vi "Init Message Transport Data Binding.vi"(8 "error in (no error)":errorcluster, 9 "Control Indexes":i32[](array[numeric]), 10 "VI Refnum":refnum<vi>) -> (0 "error out":errorcluster, 3 "Message Transport Binding out":refnum<class "Message Transport Binding.lvclass">)   [LabVIEW 2016, in "Stream Mediator.lvlib" / "Message Transport Binding.lvclass"]
doc: "--\nCopyright © 2017 Composed SystemsI All rights reserved.\n\nAuthor: Jon McBee <jon.mcbee@composed.io>\n\nThis library is provided \"AS IS\" ,WITHOUT WARRANTIES OR\nCONDITIONS OF ANY KIND, either express or implied.\n\nComposed Systems -- composed.io\n\nStream 0.0.1.1\nJon McBee - Composed Systems\nCopyright (c) 2017, Composed Systems"
uses:
  <userlib>/Composed Systems/Stream/Mediator/Classes/Message Transport Binding/Message Transport Binding.lvclass
  <userlib>/Composed Systems/Stream/Mediator/Classes/Message Transport Binding/Message Transport Binding.lvclass/Message Transport Binding.ctl
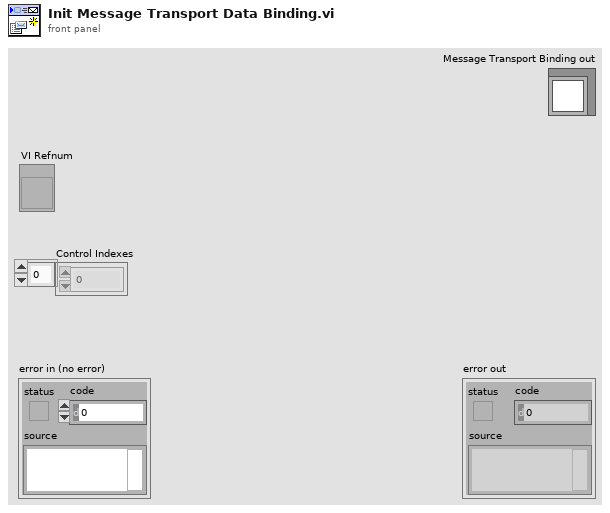
[diagram p1: front panel]
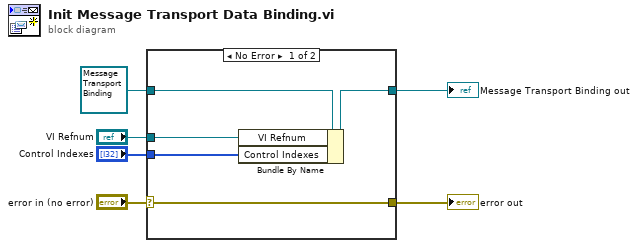
[diagram p0: block diagram]
diagram:
  n1 = case shown="No Error" "error in (no error)" {
    selector: "error in (no error)" -> [w11 w13]
    tunnel: [w11 w13] -> w5
    tunnel: [w9 w12] -> w3
    tunnel: refnum<class "Message Transport Binding.lvclass"> refnum ("Message Transport Binding in") -> [w10 w12]
    tunnel: "VI Refnum" -> [w8 _]
    tunnel: "Control Indexes" -> [w7 _]
    frame No Error {
      n2 = Bundle By Name(cluster=w10, "VI Refnum"=w8, "Control Indexes"=w7) -> (w9:refnum<class "Message Transport Binding.lvclass">)
    }
    frame Error {
    }
  }
  "error out" <- w5
  "Message Transport Binding out" <- w3
